vi "constructTopicElement.vi"(6 "firstItem? (F)":bool, 8 "error in (no error)":errorcluster, 9 "prevObjRef":refnum<vi>, 10 "clusterInfo.reference":refnum<vi>, 11 "Element in":refnum<class "Element.lvclass">) -> (0 "error out":errorcluster, 3 "Element out":refnum<class "Element.lvclass">)   [LabVIEW 2018, in "Element.lvclass"]
uses:
  Element.lvclass
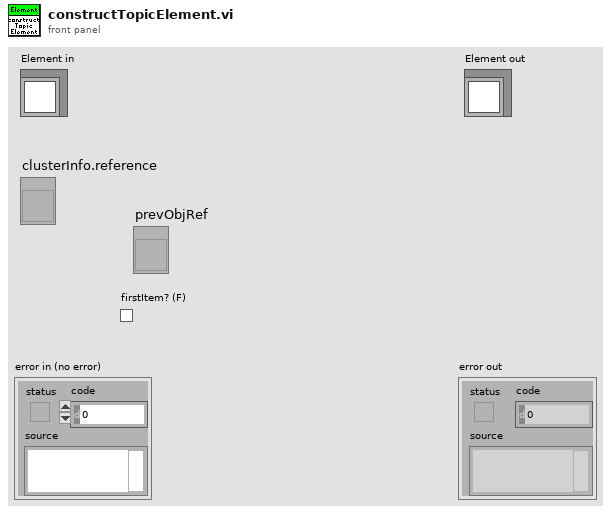
[diagram p1: front panel]
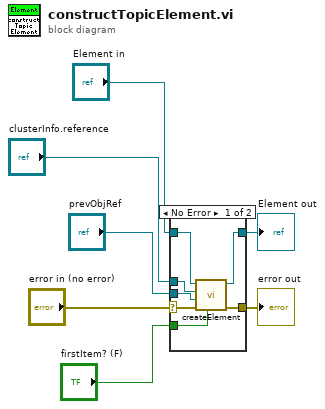
[diagram p0: block diagram]
diagram:
  n1 = case shown="No Error" "error in (no error)" {
    selector: "error in (no error)" -> [w12 w16]
    tunnel: [w11 w16] -> w6
    tunnel: [w13 w15] -> w4
    tunnel: "Element in" -> [w14 w15]
    tunnel: "clusterInfo.reference" -> [w10 _]
    tunnel: "prevObjRef" -> [w9 _]
    tunnel: "firstItem? (F)" -> [w8 _]
    frame No Error {
      n2 = call "createElement.vi"("firstItem? (F)"=w8, "error in (no error)"=w12, "prevObjRef"=w9, "clusterInfo.reference"=w10, "Element in"=w14) -> ("error out"=w11:errorcluster, "Element out"=w13:refnum<class "Element.lvclass">)  [unwired: 5 in]
    }
    frame Error {
    }
  }
  "error out" <- w6
  "Element out" <- w4
